vi "adjustLED.vi"() -> ()   [LabVIEW 2020]
uses:
  <vilib>/LabVIEW Interface for Arduino/Type Defs/Board Type.ctl
  <vilib>/LabVIEW Interface for Arduino/Type Defs/Pin Mode.ctl
  <vilib>/LabVIEW Interface for Arduino/LabVIEW Interface for Arduino.lvlib
panel:
  out "Waveform Chart":dbl(graph)
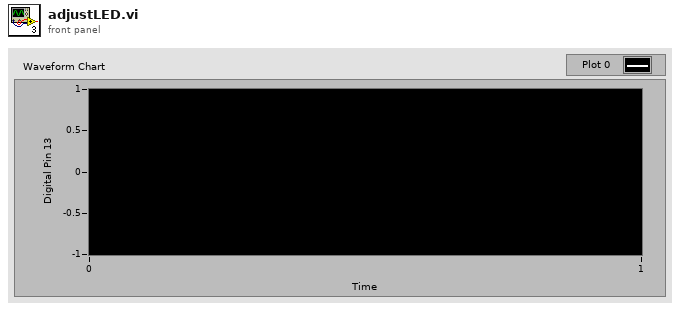
[diagram p1: front panel]
types:
  T1 = typedef "LabVIEW Interface for Arduino.lvlib/Pin Mode.ctl" = enum8{"Input", "Output"}
  T2 = typedef "LabVIEW Interface for Arduino.lvlib/Board Type.ctl" = enum16{"Uno", "Dimuelanove w/Atmega 328", "Mega 2560"}
  T3 = typedef "LabVIEW Interface for Arduino.lvlib/Arduino Resource.ctl" = cluster{"VISA resource":refnum<visa-resource-name>, "Board Type":T2, "Connection Type":enum8{"USB / Serial"}, "Bytes Per Packet (15)":u8}
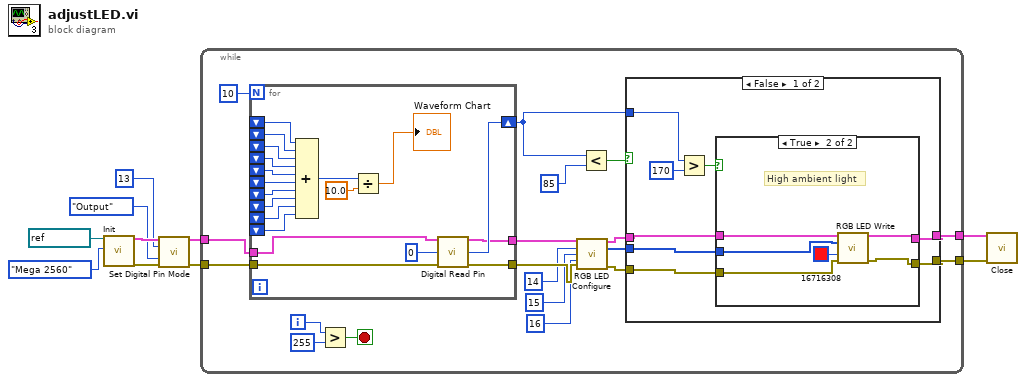
[diagram p0: block diagram]
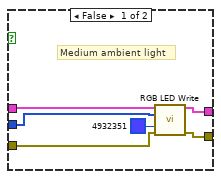
[diagram p2: hidden frame]
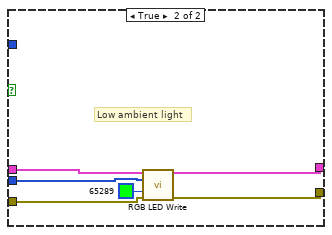
[diagram p3: hidden frame]
diagram:
  n1 = call <vilib>:"Init.vi"("VISA resource"=refnum<visa-resource-name> "COM5", "Board Type (Uno)"=Board_Type."Mega 2560") -> ("Arduino Resource"=w8:T3, "error out"=w3:errorcluster)  [unwired: 16 in]
  n2 = call <vilib>:"Set Digital Pin Mode.vi"("Arduino Resource"=w8, "Digital I/O Pin"=u8 13, "Pin Mode (Input)"=Pin_Mode."Output", "error in"=w3) -> ("Arduino Resource"=w5:T3, "error out"=w4:errorcluster)  [unwired: 10 in]
  n3 = while {
    tunnel: w5 -> [w28]
    tunnel: w4 -> [w27]
    tunnel: [w12] -> w2
    tunnel: [w11] -> w1
    i -> [w26]
    stop <- w24 stop-if-true
    n4 = for {
      N: 10 -> [_]
      tunnel: [w74] -> w22
      tunnel: [w58] -> w23
      tunnel: w28 -> [w73]
      tunnel: w27 -> [w72]
      shift-right: [w71] -> w17
      shift-left: _ -> [w70]
      shift-left: _ -> [w69]
      shift-left: _ -> [w68]
      shift-left: _ -> [w67]
      shift-left: _ -> [w66]
      shift-left: _ -> [w65]
      shift-left: _ -> [w64]
      shift-left: _ -> [w63]
      shift-left: _ -> [w62]
      shift-left: _ -> [w61]
      n5 = Compound Arithmetic op=ADD(w70, w69, w68, w67, w66, w65, w64, w63, w62, w61) -> (w59:u8)
      n6 = Divide(x=w59, y=10.0) -> (x/y=→"Waveform Chart":dbl)
      n7 = call <vilib>:"Digital Read Pin.vi"("Arduino Resource"=w73, "Digital I/O Pin (0)"=u8 0, "error in"=w72) -> ("Arduino Resource"=w58:T3, "Value"=w71:u8, "error out"=w74:errorcluster)  [unwired: 10 in]
    }
    n8 = Greater?(x=w26, y=255) -> (0:w24:bool)
    n9 = call <vilib>:"RGB LED Configure.vi"("Arduino Resource"=w23, "Red Pin"=u8 14, "Green Pin"=u8 15, "Blue Pin"=u8 16, "error in"=w22) -> ("Arduino Resource"=w15:T3, "RGB LED Pins"=w14:u8[], "error out"=w13:errorcluster)  [unwired: 8 in]
    n10 = Less?(x=w17, y=u8 85) -> (x < y?=w16:bool)
    n11 = case shown="False" w16 {
      tunnel: w17 -> [w37 _]
      tunnel: w15 -> [w34 w54]
      tunnel: w14 -> [w33 w53]
      tunnel: w13 -> [w32 w52]
      tunnel: [w31 w51] -> w12
      tunnel: [w30 w50] -> w11
      frame False {
        n12 = Greater?(x=w37, y=u8 170) -> (0:w35:bool)
        n13 = case shown="True" w35 {
          tunnel: w34 -> [w42 w48]
          tunnel: w33 -> [w41 w47]
          tunnel: w32 -> [w40 w46]
          tunnel: [w39 w45] -> w31
          tunnel: [w38 w44] -> w30
          frame False {
            # "Medium ambient light"
            n14 = call <vilib>:"RGB LED Write.vi"("Arduino Resource"=w42, "RGB LED Pins"=w41, "Color"=u32 4932351, "error in"=w40) -> ("Arduino Resource"=w39:T3, "error out"=w38:errorcluster)  [unwired: 9 in, 1 out]
          }
          frame True {
            # "High ambient light"
            n15 = call <vilib>:"RGB LED Write.vi"("Arduino Resource"=w48, "RGB LED Pins"=w47, "Color"=u32 16716308, "error in"=w46) -> ("Arduino Resource"=w45:T3, "error out"=w44:errorcluster)  [unwired: 9 in, 1 out]
          }
        }
      }
      frame True {
        # "Low ambient light"
        n16 = call <vilib>:"RGB LED Write.vi"("Arduino Resource"=w54, "RGB LED Pins"=w53, "Color"=u32 65289, "error in"=w52) -> ("Arduino Resource"=w51:T3, "error out"=w50:errorcluster)  [unwired: 9 in, 1 out]
      }
    }
  }
  n17 = call <vilib>:"Close.vi"("Arduino Resource"=w2, "error in"=w1) -> ()  [unwired: 13 in, 1 out]
